vi "CarMain_MANUAL_CONTROL.vi"() -> ()   [LabVIEW 2013]
panel:
  in  "stop":bool
  in  "Manual Motor Control":T1(ring)
  in  "Stop Array":bool[](array[boolean]) caption="Stop"
  in  "Foward Array":bool[](array[boolean]) caption="Forward"
  in  "Backward Array":bool[](array[boolean]) caption="Backward"
  in  "Turn Left Array":bool[](array[boolean]) caption="Turn Left"
  in  "Turn Right Array":bool[](array[boolean]) caption="Turn Right"
  # "This template is used test your car MANUALLY (by selecting \n\"turn right\", \"go forward\", etc.) This will NOT be the final template\nthat you use in the project, but it will be useful at the BEGINNING of the project. \nOnce you attach your myDAQ with your four digital outputs to\nthe H-bridge and connect the H-bridge to the motors, you can use\nthis template to make sure that your arrays are set correctly. For example,\nMANUALLY set your car to \"go forward\" and make sure that when you do, \nyour car actaully goes forward. Make sure these arrays are set properly before\nyou move onto the digital (boolean) logic that is used  to get your car to move on its own."
  # "note 1: ONE ARRAY = 4 DIGITAL OUTPUTS (4 bits)\nnote 2: This template contains NO inputs, you manually\n              set the condition (i.e. forward, stop, ...) and the \n              one DAQ on the block diagram will output \n              the specified array.\nnote 3: Go to the block diagram, double click on the green array\n             blocks to see for yourself that these \"4 dot\" arrays on this\n             front pannel corespond with the blocks"
  # "These are the output arrays. Click\nthe dot (it should turn black) to make\nthe array value a one. A light gray\ndot represents a zero."
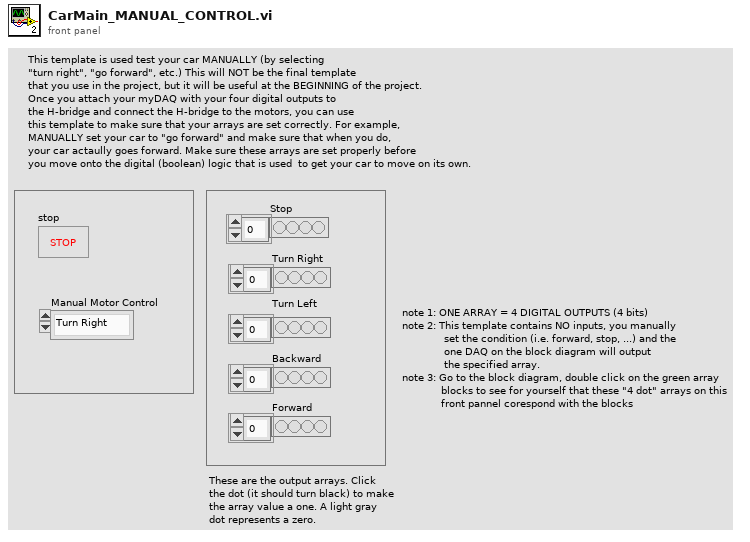
[diagram p1: front panel]
types:
  T1 = enum16{"Turn Right", "Turn Left", "Backward", "Forward", "Stop"}
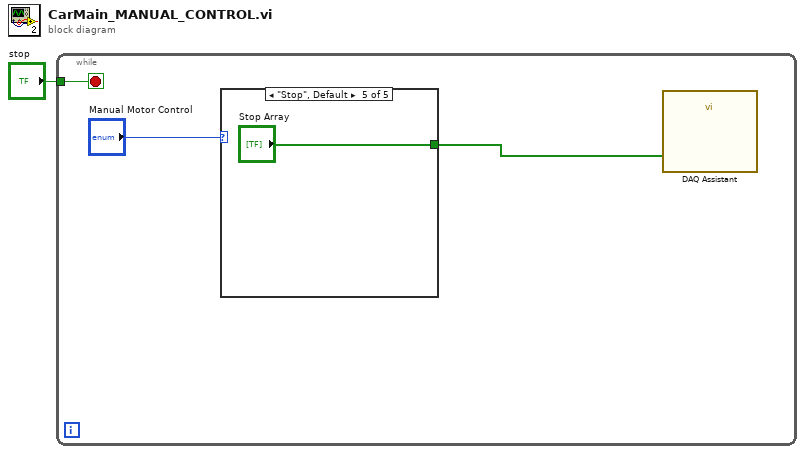
[diagram p0: block diagram]
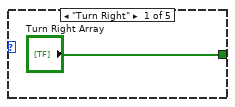
[diagram p2: hidden frame]
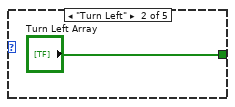
[diagram p3: hidden frame]
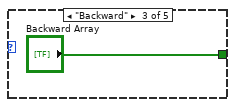
[diagram p4: hidden frame]
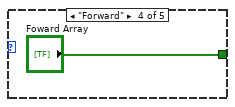
[diagram p5: hidden frame]
diagram:
  n1 = while {
    tunnel: "stop" -> [w3]
    stop <- w3 stop-if-true
    n2 = case shown="\"Stop\", Default" "Manual Motor Control" {
      tunnel: ["Turn Right Array" "Turn Left Array" "Backward Array" "Foward Array" "Stop Array"] -> w2
      frame "Turn Right" {
      }
      frame "Turn Left" {
      }
      frame "Backward" {
      }
      frame "Forward" {
      }
      frame "Stop", Default {
      }
    }
    n3 = call "DAQ Assistant"("data"=w2) -> ()  [unwired: 17 in, 2 out]
  }
